vi "Slots.vi"() -> ()   [LabVIEW 2021]
uses:
  <vilib>/numeric/Random Number (Range) U64.vi
  <vilib>/numeric/sub_Random U32.vi
panel:
  out "3":picture
  out "2":picture
  out "1":picture
  in  "?":bool
  out "Bet":dbl
  in  "?":bool
  out "Credit":dbl
  in  "?":bool
  in  "?":bool
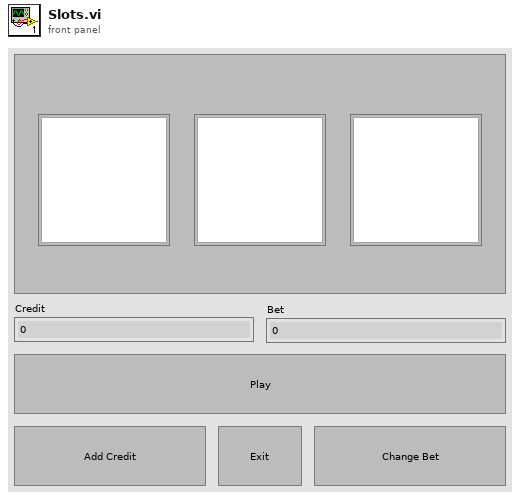
[diagram p1: front panel]
types:
  T1 = enum16{"Init", "Exit", "Wait", "AddCredit", "Play", "Win", "Double", "ChangeCredit"}
  T2 = typedef "imagedata.ctl" = cluster{"image type":i32, "image depth":i32, "image":u8[], "mask":u8[], "colors":u32[], "Rectangle":cluster{"left":i16, "top":i16, "right":i16, "bottom":i16}}
  T3 = enum16{"Left Button", "Center Button", "Right Button", "Window Close"}
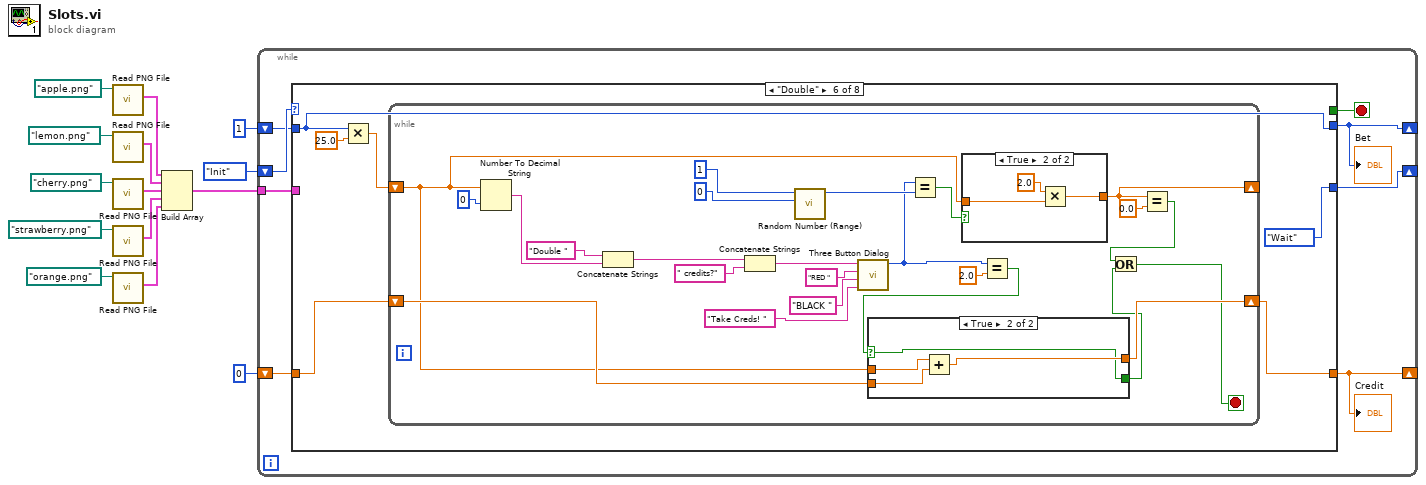
[diagram p0: block diagram]
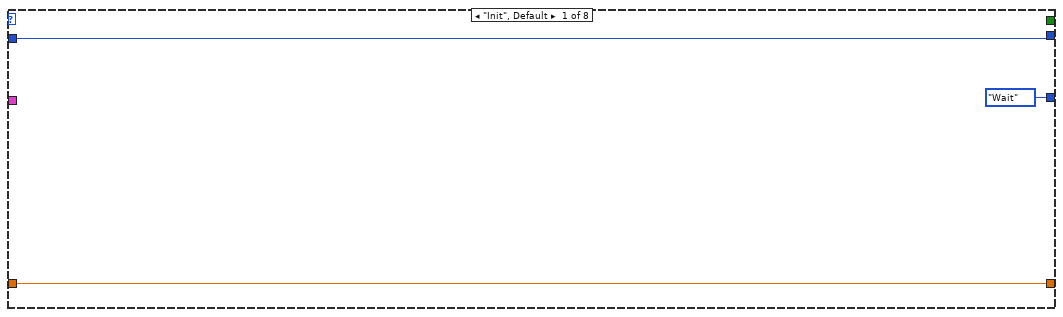
[diagram p2: hidden frame]
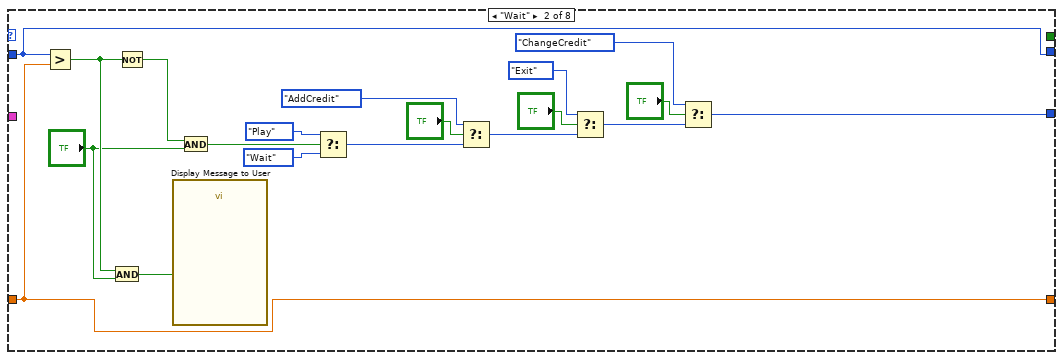
[diagram p3: hidden frame]
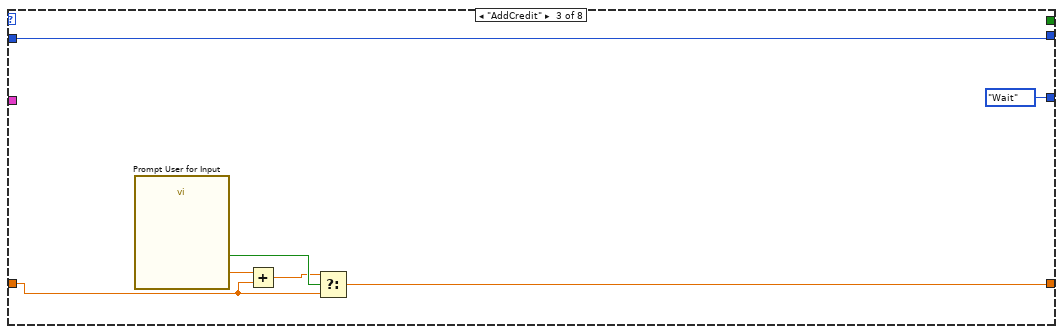
[diagram p4: hidden frame]
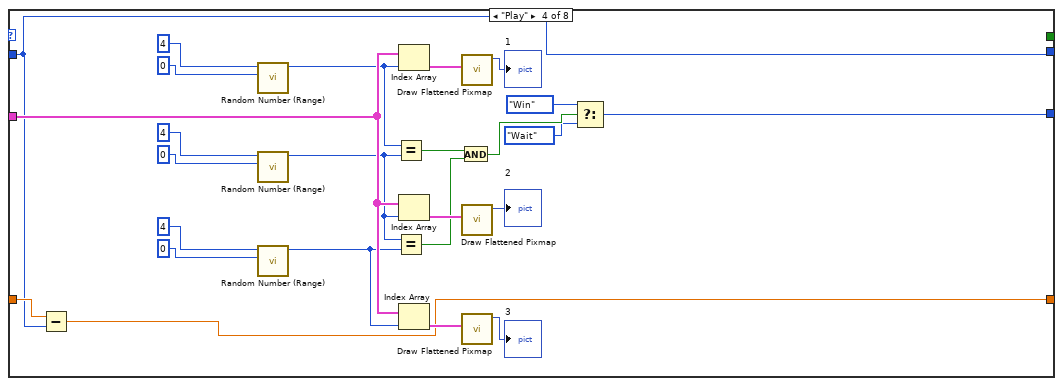
[diagram p5: hidden frame]
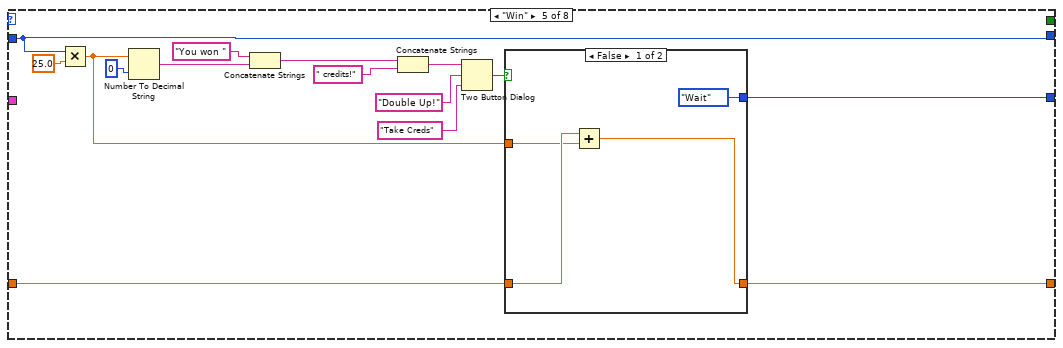
[diagram p6: hidden frame]
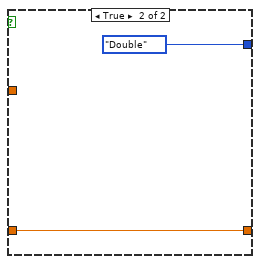
[diagram p7: hidden frame]
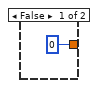
[diagram p9: hidden frame]
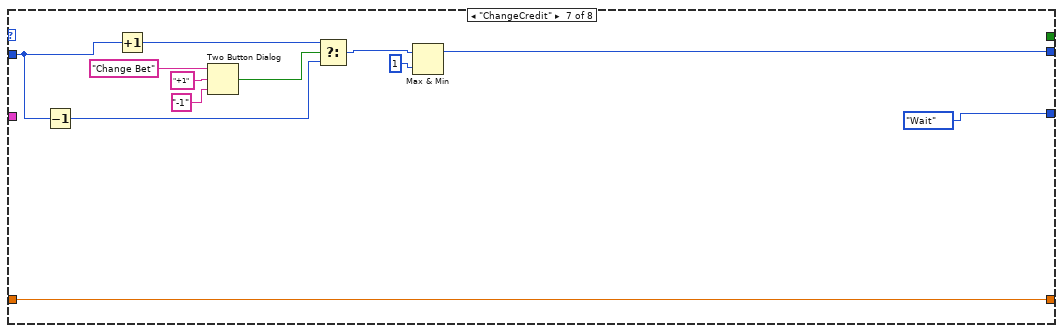
[diagram p10: hidden frame]
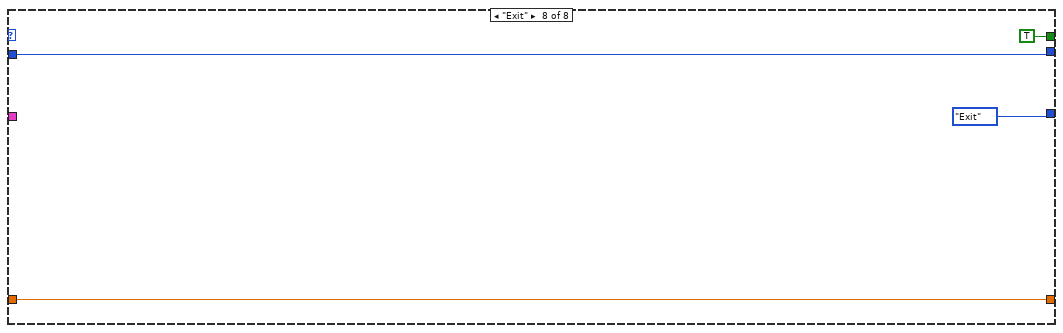
[diagram p11: hidden frame]
diagram:
  n1 = call <vilib>:"Read PNG File.vi"("path to PNG file"=path "apple.png") -> ("image data"=w6:T2)  [unwired: 8 in, 2 out]
  n2 = call <vilib>:"Read PNG File.vi"("path to PNG file"=path "lemon.png") -> ("image data"=w5:T2)  [unwired: 8 in, 2 out]
  n3 = call <vilib>:"Read PNG File.vi"("path to PNG file"=path "cherry.png") -> ("image data"=w4:T2)  [unwired: 8 in, 2 out]
  n4 = call <vilib>:"Read PNG File.vi"("path to PNG file"=path "strawberry.png") -> ("image data"=w3:T2)  [unwired: 8 in, 2 out]
  n5 = call <vilib>:"Read PNG File.vi"("path to PNG file"=path "orange.png") -> ("image data"=w2:T2)  [unwired: 8 in, 2 out]
  n6 = Build Array(w6, w5, w4, w3, w2) -> (w1:T2[])
  n7 = while {
    shift-right: [w21] -> _
    shift-left: T1."Init" ("Enum") -> [w22]
    shift-right: [w17] -> _
    shift-left: 0 -> [w19]
    shift-right: [w16] -> _
    shift-left: 1 -> [w18]
    tunnel: w1 -> [w15]
    stop <- w20 stop-if-true
    n8 = case shown="\"Double\"" w22 {
      tunnel: [T1."Wait" ("Enum") w33 T1."Wait" ("Enum") w52 w80 T1."Wait" ("Enum") T1."Wait" ("Enum") T1."Exit" ("Enum")] -> w21
      tunnel: [_ _ _ _ _ _ _ TRUE] -> w20
      tunnel: w19 -> [w24 w32 w49 w63 w79 w100 w149 w152]
      tunnel: [w24 w32 w47 w62 w77 w99 w149 w152] -> w17
      tunnel: w18 -> [w23 w31 w46 w61 w87 w102 w144 w151]
      tunnel: [w23 w31 w46 w61 w87 w102 w139 w151] -> w16
      tunnel: w15 -> [_ _ _ w68 _ _ _ _]
      frame "Init", Default {
      }
      frame "Wait" {
        n9 = Greater?(x=w31, y=w32) -> (0:w28:bool)
        n10 = And(x=w28, y="?") -> (x .and. y?=w30:bool)
        n11 = Not(x=w28) -> (.not. x?=w29:bool)
        n12 = call "Display Message to User"("Enable"=w30) -> ()  [unwired: 9 in, 2 out]
        n13 = And(x=w29, y="?") -> (x .and. y?=w26:bool)
        n14 = Select(t=T1."Play" ("Enum"), s=w26, f=T1."Wait" ("Enum")) -> (s? t:f=w39:T1)
        n15 = Select(t=T1."AddCredit" ("Enum"), s="?", f=w39) -> (s? t:f=w38:T1)
        n16 = Select(t=T1."Exit" ("Enum"), s="?", f=w38) -> (s? t:f=w34:T1)
        n17 = Select(t=T1."ChangeCredit" ("Enum"), s="?", f=w34) -> (s? t:f=w33:T1)
      }
      frame "AddCredit" {
        n18 = call "Prompt User for Input"() -> ("Credit"=w50:dbl, "OK"=w51:bool)  [unwired: 17 in, 1 out]
        n19 = Add(x=w50, y=w49) -> (x+y=w48:dbl)
        n20 = Select(t=w48, s=w51, f=w49) -> (s? t:f=w47:dbl)
      }
      frame "Play" {
        n21 = Subtract(x=w63, y=w61) -> (x-y=w62:dbl)
        n22 = call-poly <vilib>:"Random Number (Range).vi"("lower bound (0)"=u64 0, "upper bound (100)"=u64 4) -> ("number"=w60:u64)  [unwired: 9 in]
        n23 = call-poly <vilib>:"Random Number (Range).vi"("lower bound (0)"=u64 0, "upper bound (100)"=u64 4) -> ("number"=w59:u64)  [unwired: 9 in]
        n24 = call-poly <vilib>:"Random Number (Range).vi"("lower bound (0)"=u64 0, "upper bound (100)"=u64 4) -> ("number"=w58:u64)  [unwired: 9 in]
        n25 = Equal?(x=w60, y=w59) -> (x = y?=w57:bool)
        n26 = Equal?(x=w59, y=w58) -> (x = y?=w56:bool)
        n27 = Index Array(array=w68, index=w60) -> (element=w76:T2)
        n28 = Index Array(array=w68, index=w59) -> (element=w65:T2)
        n29 = Index Array(array=w68, index=w58) -> (element=w64:T2)
        n30 = And(x=w57, y=w56) -> (x .and. y?=w55:bool)
        n31 = call <vilib>:"Draw Flattened Pixmap.vi"("image data"=w76) -> ("new picture"=→"1":picture)  [unwired: 8 in]
        n32 = call <vilib>:"Draw Flattened Pixmap.vi"("image data"=w65) -> ("new picture"=→"2":picture)  [unwired: 8 in]
        n33 = call <vilib>:"Draw Flattened Pixmap.vi"("image data"=w64) -> ("new picture"=→"3":picture)  [unwired: 8 in]
        n34 = Select(t=T1."Win" ("Enum"), s=w55, f=T1."Wait" ("Enum")) -> (s? t:f=w52:T1)
      }
      frame "Win" {
        n35 = Multiply(x=w87, y=25.0) -> (x*y=w78:dbl)
        n36 = Number To Decimal String(number=w78, width (-)=i16 0) -> (decimal integer string=w85:string)
        n37 = Concatenate Strings("You won " ("message"), w85) -> (w84:string)
        n38 = Concatenate Strings(w84, " credits!" ("message")) -> (w82:string)
        n39 = Two Button Dialog(message=w82, 1:"Take Creds" ("F button name (\"Cancel\")"), 2:"Double Up!" ("T button name (\"OK\")")) -> (T button?=w81:bool)
        n40 = case shown="False" w81 {
          tunnel: [T1."Wait" ("Enum") T1."Double" ("Enum")] -> w80
          tunnel: w79 -> [w95 w96]
          tunnel: w78 -> [w94 _]
          tunnel: [w93 w96] -> w77
          frame False {
            n41 = Add(x=w95, y=w94) -> (x+y=w93:dbl)
          }
          frame True {
          }
        }
      }
      frame "Double" {
        n42 = Multiply(x=w102, y=25.0) -> (x*y=w101:dbl)
        n43 = while {
          shift-right: [w110] -> _
          shift-left: w101 -> [w107]
          shift-right: [w106] -> w99
          shift-left: w100 -> [w108]
          stop <- w105 stop-if-true
          n44 = Number To Decimal String(number=w107, width (-)=i16 0) -> (decimal integer string=w117:string)
          n45 = Concatenate Strings("Double " ("message"), w117) -> (w118:string)
          n46 = Concatenate Strings(w118, " credits?" ("message")) -> (w113:string)
          n47 = call-poly <vilib>:"Random Number (Range).vi"("lower bound (0)"=u64 0, "upper bound (100)"=u64 1) -> ("number"=w121:u64)  [unwired: 9 in]
          n48 = call <vilib>:"Three Button Dialog.vi"("Right Button Text (\"Cancel\")"="Take Creds! " ("message"), "Center Button Text (\"No\")"="BLACK " ("message"), "Left Button Text (\"Yes\")"="RED " ("message"), "message"=w113) -> ("Which Button?"=w120:T3)  [unwired: 7 in]
          n49 = Equal?(x=w120, y=w121) -> (x = y?=w119:bool)
          n50 = case shown="True" w119 {
            tunnel: w107 -> [_ w136]
            tunnel: [0 w135] -> w110
            frame False {
            }
            frame True {
              n51 = Multiply(x=2.0 ("y"), y=w136) -> (x*y=w135:dbl)
            }
          }
          n52 = Equal?(x=w120, y=2.0) -> (x = y?=w109:bool)
          n53 = case shown="True" w109 {
            selector: w109 -> [w128 w130]
            tunnel: w108 -> [w129 w132]
            tunnel: w107 -> [_ w133]
            tunnel: [w129 w131] -> w106
            tunnel: [w128 w130] -> w104
            frame False {
            }
            frame True {
              n54 = Add(x=w133, y=w132) -> (x+y=w131:dbl)
            }
          }
          n55 = Equal?(x=w110, y=0.0) -> (x = y?=w111:bool)
          n56 = Or(x=w111, y=w104) -> (x .or. y?=w105:bool)
        }
      }
      frame "ChangeCredit" {
        n57 = Decrement(x=w144) -> (x-1=w143:i32)
        n58 = Increment(x=w144) -> (x+1=w142:i32)
        n59 = Two Button Dialog(message="Change Bet", 1:"-1", 2:"+1") -> (T button?=w145:bool)
        n60 = Select(t=w142, s=w145, f=w143) -> (s? t:f=w140:i32)
        n61 = Max & Min(x=w140, y=1) -> (max(x,y)=w139:i32)  [unwired: 1 out]
      }
      frame "Exit" {
      }
    }
    "Credit" <- w17
    "Bet" <- w16
  }
